vi "Test_Sin acq point.vi"() -> ()   [LabVIEW 2015]
panel:
  out "Init Data Out":u16[](array[numeric])
  out "Total Pixel/Line":dbl
  out "Average Per Pixel Dis.":dbl[][](graph)
  out "Total Average Per Pixel":dbl[](array[numeric])
  in  "Scanning Speed":dbl=2000.0
  in  "Sample Rate":dbl=120000000.0 format="%#_6p"
  in  "Fill Fraction":dbl=0.85
  in  "Effecte Pixel/Line":dbl=512.0
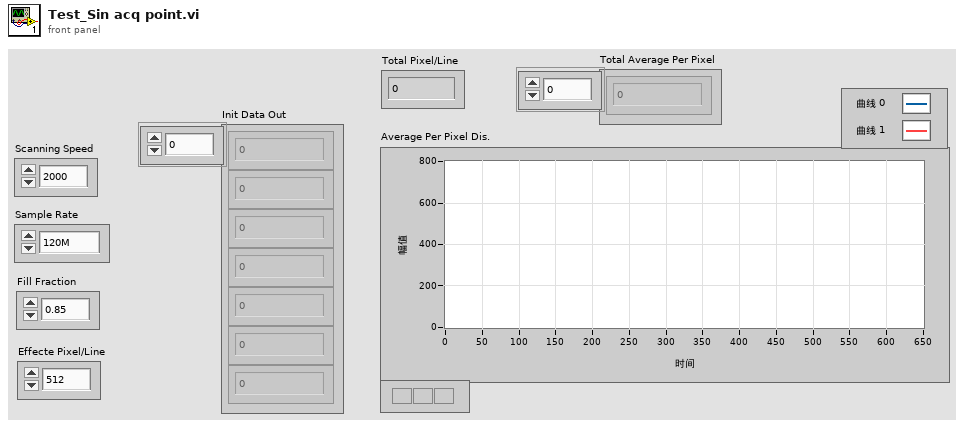
[diagram p1: front panel]
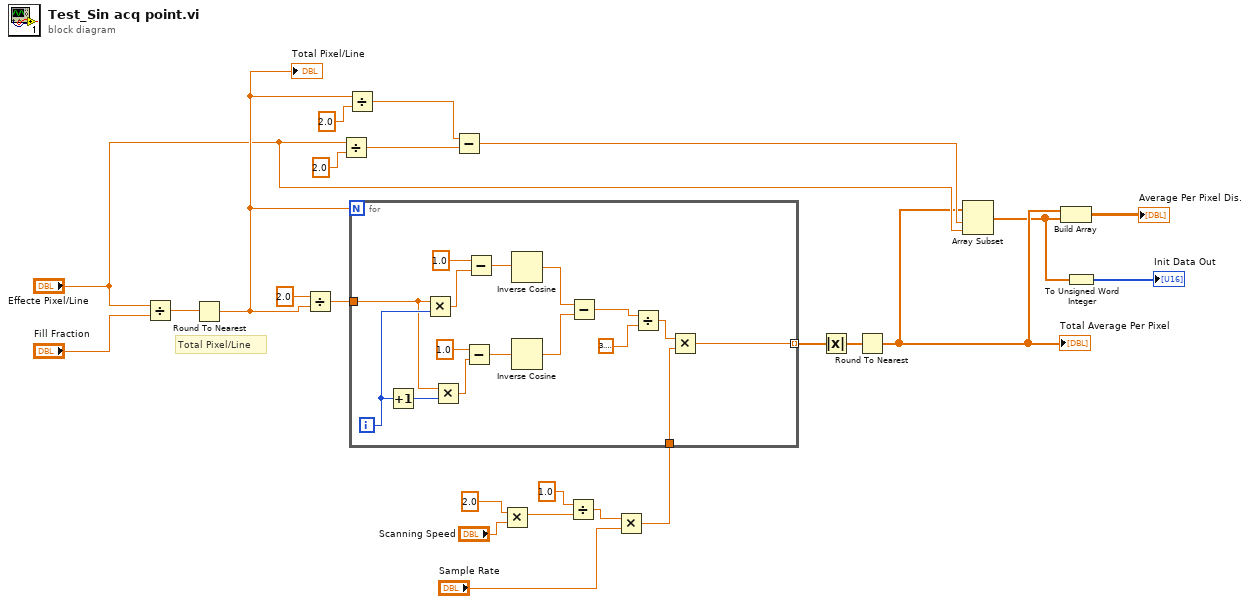
[diagram p0: block diagram]
diagram:
  # "Total Pixel/Line"
  n1 = Divide(x="Effecte Pixel/Line", y="Fill Fraction") -> (x/y=w23:dbl)
  n2 = Round To Nearest(number=w23) -> (nearest integer value=w11:dbl)
  "Total Pixel/Line" <- w11
  n3 = Divide(x=2.0, y=w11) -> (x/y=w21:dbl)
  n4 = Divide(x="Effecte Pixel/Line", y=2.0) -> (x/y=w6:dbl)
  n5 = Divide(x=w11, y=2.0) -> (x/y=w9:dbl)
  n6 = Subtract(x=w9, y=w6) -> (x-y=w8:dbl)
  n7 = Multiply(x=2.0, y="Scanning Speed") -> (x*y=w15:dbl)
  n8 = Divide(x=1.0, y=w15) -> (x/y=w14:dbl)
  n9 = Multiply(x=w14, y="Sample Rate") -> (x*y=w19:dbl)
  n10 = for {
    N: w11 -> [_]
    tunnel: w21 -> [w31]
    tunnel: w19 -> [w26]
    tunnel: [w25] -> w17 mode=indexing
    i -> [w34]
    n11 = Increment(x=w34) -> (x+1=w33:i32)
    n12 = Multiply(x=w31, y=w34) -> (x*y=w36:dbl)
    n13 = Multiply(x=w31, y=w33) -> (x*y=w32:dbl)
    n14 = Subtract(x=1.0, y=w32) -> (x-y=w30:dbl)
    n15 = Subtract(x=1.0, y=w36) -> (x-y=w37:dbl)
    n16 = Inverse Cosine(1:w37) -> (0:w40:dbl)
    n17 = Inverse Cosine(1:w30) -> (0:w39:dbl)
    n18 = Subtract(x=w40, y=w39) -> (x-y=w29:dbl)
    n19 = Divide(x=w29, y=3.141592653589793) -> (x/y=w27:dbl)
    n20 = Multiply(x=w27, y=w26) -> (x*y=w25:dbl)
  }
  n21 = Absolute Value(x=w17) -> (abs(x)=w12:dbl[])
  n22 = Round To Nearest(number=w12) -> (nearest integer value=w4:dbl[])
  "Total Average Per Pixel" <- w4
  n23 = Array Subset(array=w4, index=w8, length="Effecte Pixel/Line") -> (w2:dbl[])
  n24 = Build Array(w4, w2) -> (→"Average Per Pixel Dis.":dbl[][])
  n25 = To Unsigned Word Integer(number=w2) -> (unsigned 16bit integer=→"Init Data Out":u16[])
